vi "Network Send.vi"(8 "error in (no error)":errorcluster, 10 "Target IP Address":string="localhost", 11 "Electrophysiology in":refnum<class "Electrophysiology.lvclass">) -> (0 "error out":errorcluster, 3 "Electrophysiology out":refnum<class "Electrophysiology.lvclass">)   [LabVIEW 2010, in "Electrophysiology.lvclass"]
uses:
  Electrophysiology.lvclass
  Electrophysiology.lvclass/Electrophysiology.ctl
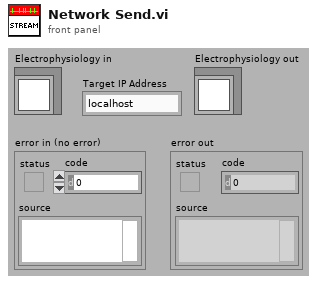
[diagram p1: front panel]
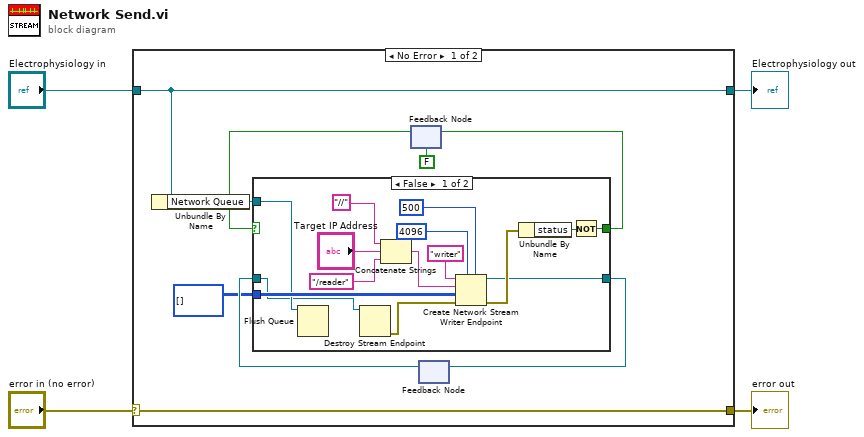
[diagram p0: block diagram]
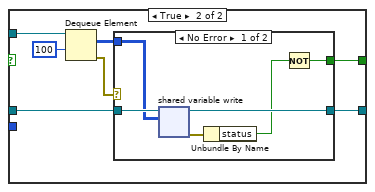
[diagram p2: hidden frame]
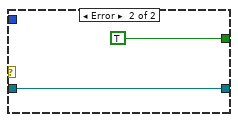
[diagram p3: hidden frame]
diagram:
  n1 = case shown="No Error" "error in (no error)" {
    selector: "error in (no error)" -> [w13 w45]
    tunnel: [w13 w45] -> w3
    tunnel: [w6 w44] -> w1
    tunnel: "Electrophysiology in" -> [w6 w44]
    frame No Error {
      n2 = Unbundle By Name(w6) -> ("Network Queue"=w5:refnum<queue>)
      n3 = feedback #1(FALSE) -> (w11:bool)
      n4 = feedback #2() -> (w9:refnum<k21>)  [unwired: 1 in]
      n5 = case shown="False" w11 {
        tunnel: i32[][] [] -> [w25 _]
        tunnel: [w21 w29] -> w12
        tunnel: [w23 w32] -> w10
        tunnel: w9 -> [w16 w34]
        tunnel: w5 -> [w17 w35]
        frame False {
          n6 = Flush Queue(queue=w17) -> ()  [unwired: 1 in, 3 out]
          n7 = Destroy Stream Endpoint(11:w16) -> (0:w15:errorcluster)  [unwired: 1 in]
          n8 = Concatenate Strings("//" ("reader url"), "Target IP Address", "/reader" ("string")) -> (w14:string)
          n9 = Create Network Stream Writer Endpoint(5:500 ("timeout in ms (-1)"), 7:4096 ("writer buffer size"), 8:w15, 9:w25, 10:w14, 11:"writer" ("writer name")) -> (0:w24:errorcluster, 3:w23:refnum<k21>)
          n10 = Unbundle By Name(w24) -> ("status"=w22:bool)
          n11 = Not(x=w22) -> (.not. x?=w21:bool)
        }
        frame True {
          n12 = Dequeue Element(queue=w35, timeout in ms (-1)=100) -> (element=w33:i32[][], error out=w30:errorcluster)  [unwired: 1 in, 2 out]
          n13 = case shown="No Error" w30 {
            tunnel: w34 -> [w41 w43]
            tunnel: w33 -> [w40 _]
            tunnel: [w39 w43] -> w32
            tunnel: [w36 TRUE] -> w29
            frame No Error {
              n14 = shared-variable-write(w41, w40) -> (w39:refnum<k21>, w38:errorcluster)  [unwired: 2 in, 1 out]
              n15 = Unbundle By Name(w38) -> ("status"=w37:bool)
              n16 = Not(x=w37) -> (.not. x?=w36:bool)
            }
            frame Error {
            }
          }
        }
      }
      n17 = feedback-in #1(w12) -> ()
      n18 = feedback-in #2(w10) -> ()
    }
    frame Error {
    }
  }
  "error out" <- w3
  "Electrophysiology out" <- w1
